vi "Synergy - Position-Position.vi"(10 "Angle for Synergy analysis":dbl[][](array[numeric]), 11 "Position (output)":dbl[][](array[numeric])) -> (2 "Synergy Graph":i32[][](array[numeric]), 3 "Synergy%":i32[][](array[numeric]))   [LabVIEW 2020]
uses:
  <vilib>/Analysis/NI_AALPro.lvlib
panel:
  out "Shoulder Angle Zaxis":dbl[](graph)
  out "WristY-Shoulder Angle Zaxis graph 4":i32[](graph)
  out "WristY-Shoulder AngleZ opposite direction % 4":i32
  out "WristY-Shoulder Angle Zaxis same direction %4":i32
  out "WristY-Shoulder Angle Zaxis graph 3":i32[](graph)
  out "WristY-Shoulder AngleZ opposite direction % 3":i32
  out "WristY-Shoulder Angle Zaxis same direction % 3":i32
  out "WristX-Shoulder Angle Zaxis graph 2":i32[](graph)
  out "WristX-Shoulder Angle Zaxis opposite direction % 2":i32
  out "WristX-Shoulder Angle Zaxis same direction % 2":i32
  out "Wrist Y Tags 2":i32[](array[numeric])
  out "WristY-Elbow Angle Zaxis graph 2":i32[](graph)
  out "WristY-Elbow AngleZ opposite direction % 2":i32
  out "WristY-Elbow Angle Zaxis same direction % 2":i32
  out "WristY-ElbowY graph 2":i32[](graph)
  out "WristY-ElbowY opposite direction % 2":i32
  out "WristY-ElbowY same direction % 2":i32
  out "WristY-ElbowX graph 2":i32[](graph)
  out "WristY-ElbowX opposite direction % 2":i32
  out "WristY-ElbowX same direction % 2":i32
  out "WristY-ShoulderY graph 2":i32[](graph)
  out "WristY-ShouldeY opposite direction % 2":i32
  out "WristY-ShouldeY same direction % 2":i32
  out "WristY-ShoulderX graph 2":i32[](graph)
  out "WristY-ShouldeX opposite direction % 2":i32
  out "WristY- ShoulderX same direction % 2":i32
  out "Elbow Angle Zaxis":dbl[](graph)
  out "WristY-Elbow Angle Zaxis graph":i32[](graph)
  out "WristY-Elbow AngleZ opposite direction %":i32
  out "WristY-Elbow Angle Zaxis same direction %":i32
  out "WristX-Elbow Angle Zaxis graph":i32[](graph)
  out "WristX-Elbow Angle Zaxis opposite direction %":i32
  out "WristX-Elbow Angle Zaxis same direction %":i32
  out "Array 2":i32[](array[numeric])
  out "WristX derivative":dbl[](graph)
  out "WristX":dbl[](graph)
  out "WristX cropped region":dbl[](graph)
  out "WristY-ElbowY graph":i32[](graph)
  out "WristY-ElbowY opposite direction %":i32
  out "WristY-ElbowY same direction %":i32
  out "WristY-ElbowX graph":i32[](graph)
  out "WristY-ElbowX opposite direction %":i32
  out "WristY-ElbowX same direction %":i32
  out "WristY-ShoulderY graph":i32[](graph)
  out "WristY-ShouldeY opposite direction %":i32
  out "WristY-ShouldeY same direction %":i32
  out "WristY-ShoulderX graph":i32[](graph)
  out "WristY-ShouldeX opposite direction %":i32
  out "WristY- ShoulderX same direction %":i32
  out "WristX-ElbowY graph":i32[](graph)
  out "WristX-ElbowY opposite direction %":i32
  out "WristX-ElbowY same direction %":i32
  out "WristX-ElbowX graph":i32[](graph)
  out "WristX-ElbowX opposite direction %":i32
  out "WristX-ElbowX same direction %":i32
  out "WristX-ShoulderY graph":i32[](graph)
  out "WristX-ShouldeY opposite direction %":i32
  out "WristX-ShouldeY same direction %":i32
  out "Shoulder Y to derivate":dbl[](array[numeric])
  out "WristX-ShoulderX graph":i32[](graph)
  out "WristX-ShouldeX opposite direction %":i32
  out "WristX-ShouldeX same direction %":i32
  out "Wrist X to derivate":dbl[](array[numeric])
  out "Wrist X to graph":dbl[](array[numeric])
  out "Shoulder X to derivate":dbl[](array[numeric])
  out "Shoulder X":dbl[](array[numeric])
  out "Wrist Y Tags":i32[](array[numeric])
  out "Wrist X Tags":i32[](array[numeric])
  out "?":dbl[](graph)
  out "Elbow Y":dbl[](graph)
  out "Elbow X":dbl[](graph)
  out "Shoulder Y":dbl[](graph)
  out "?":dbl[](graph)
  # "0 WristX-ShoulderX - same direction\n1 WristX-ShoulderX - opposite direction\n2 WristX-ShoulderY - same direction\n3 - WristX-ShoulderY - opposite direction\n4 WristX-ElbowX - same direction\n5 - WristX-ElbowX - opposite direction\n6 WristX-ElbowY - same direction\n7 - WristX-ElbowY - opposite direction\n8 WristY (up)-ShoulderX - same direction\n9 WristY (up)-ShoulderX - opposite direction\n10 WristY (up)-ShoulderY - same direction\n11 - WristY (up)-ShoulderY - opposite direction\n12 WristY (up)-ElbowX - same direction\n13 - WristY (up)-ElbowX - opposite direction\n14 WristY (up)-ElbowY - same direction\n15 - WristY (up)-ElbowY - opposite direction\n16 WristX-Elbow angle Zaxis - same direction\n17 WristX-Elbow angle Zaxis- opposite direction\n18 WristY (up)-Elbow angle Zaxis - same direction\n19 - WristY (up)-Elbow angle Zaxis - opposite direction\n20 WristY (down)-ShoulderX - same direction\n21 WristY (down)-ShoulderX - opposite direction\n22 WristY (down)-ShoulderY - same direction\n23 - WristY (down)-ShoulderY - opposite direction\n24 WristY (down)-ElbowX - same direction\n25 - WristY (down)-ElbowX - opposite direction\n26 WristY (down)-ElbowY - same direction\n27 - WristY (down)-ElbowY - opposite direction\n28 WristY (down)-Elbow angle Zaxis - same direction\n29 - WristY (down)-Elbow angle Zaxis - opposite direction\n30 WristX-Shoulder angle Zaxis - same direction\n31 WristX-Shoulder angle Zaxis- opposite direction\n32 WristY (up)-Shoulder angle Zaxis - same direction\n33 - WristY (up)-Shoulder angle Zaxis - opposite direction\n34 WristY (down)-Shoulder angle Zaxis - same direction\n35 - WristY (down)-Shoulder angle Zaxis - opposite direction"
  # "wrist Y"
  # "wrist X"
  # "derivative"
  # "derivative"
  # "Shoulder X"
  # "Shoulder Y"
  # "Shoulder Z"
  # "Elbow X"
  # "Elbow Y"
  # "Elbow Z"
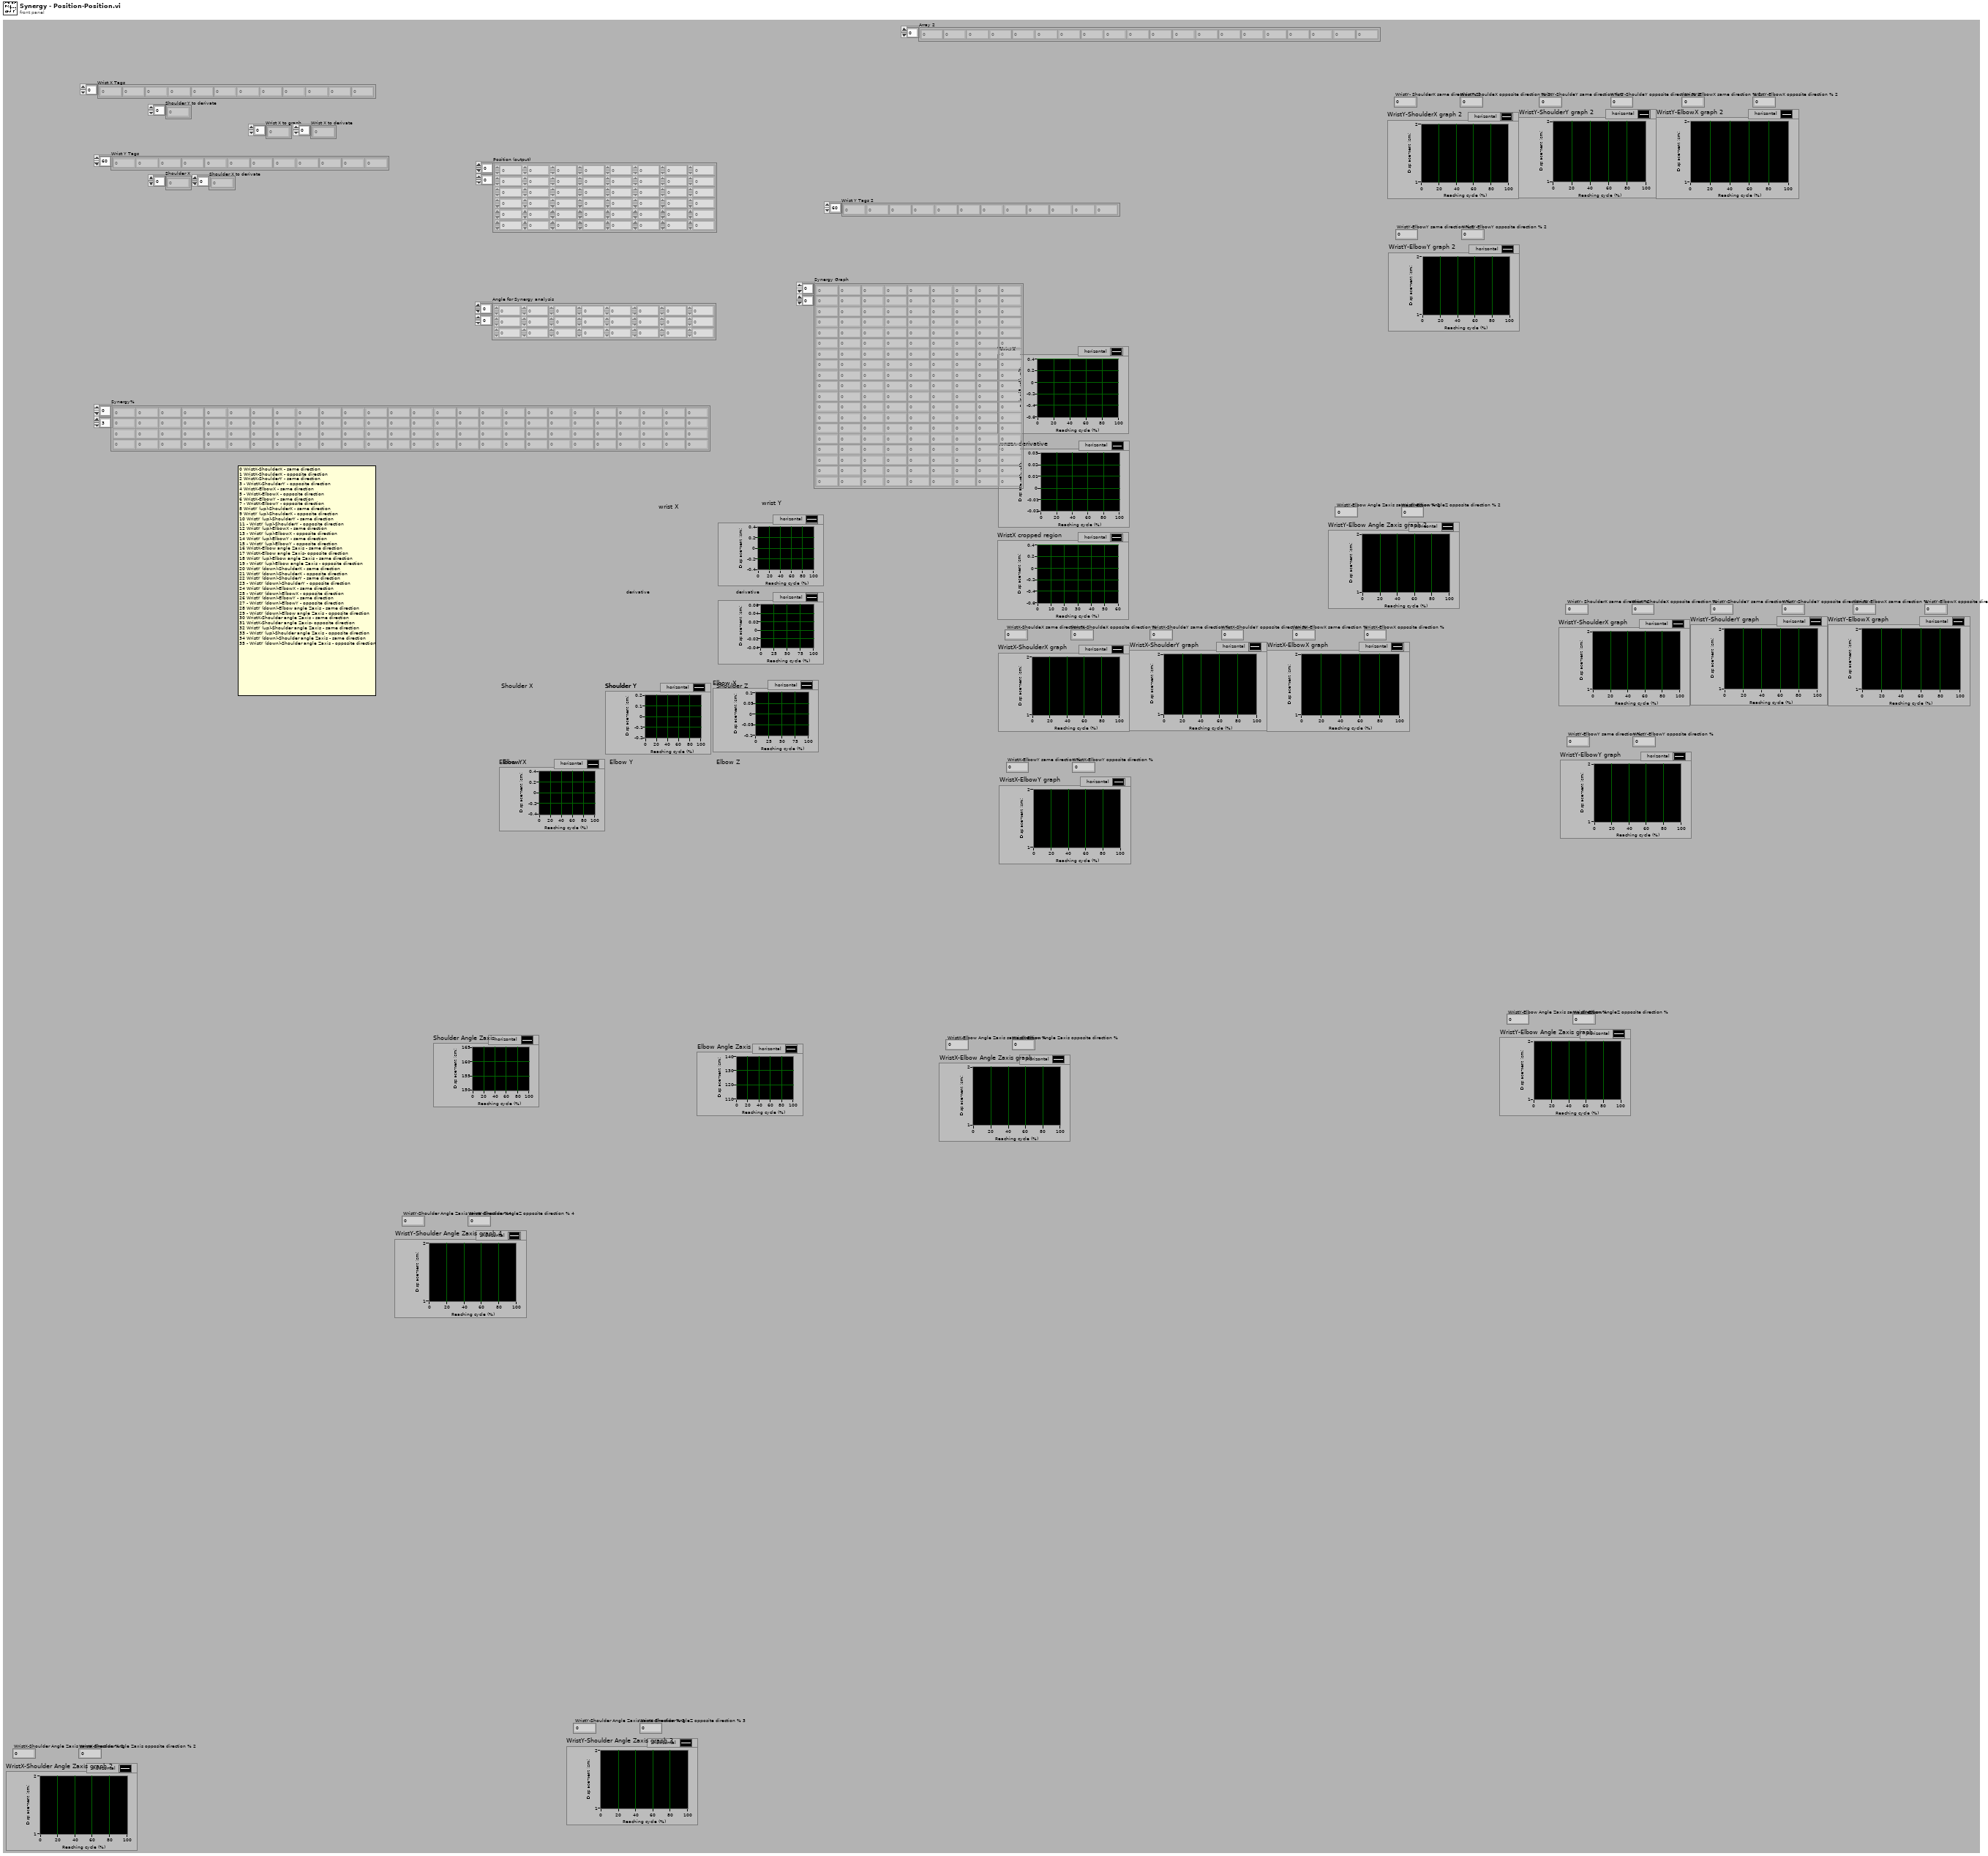
[diagram p1: front panel]
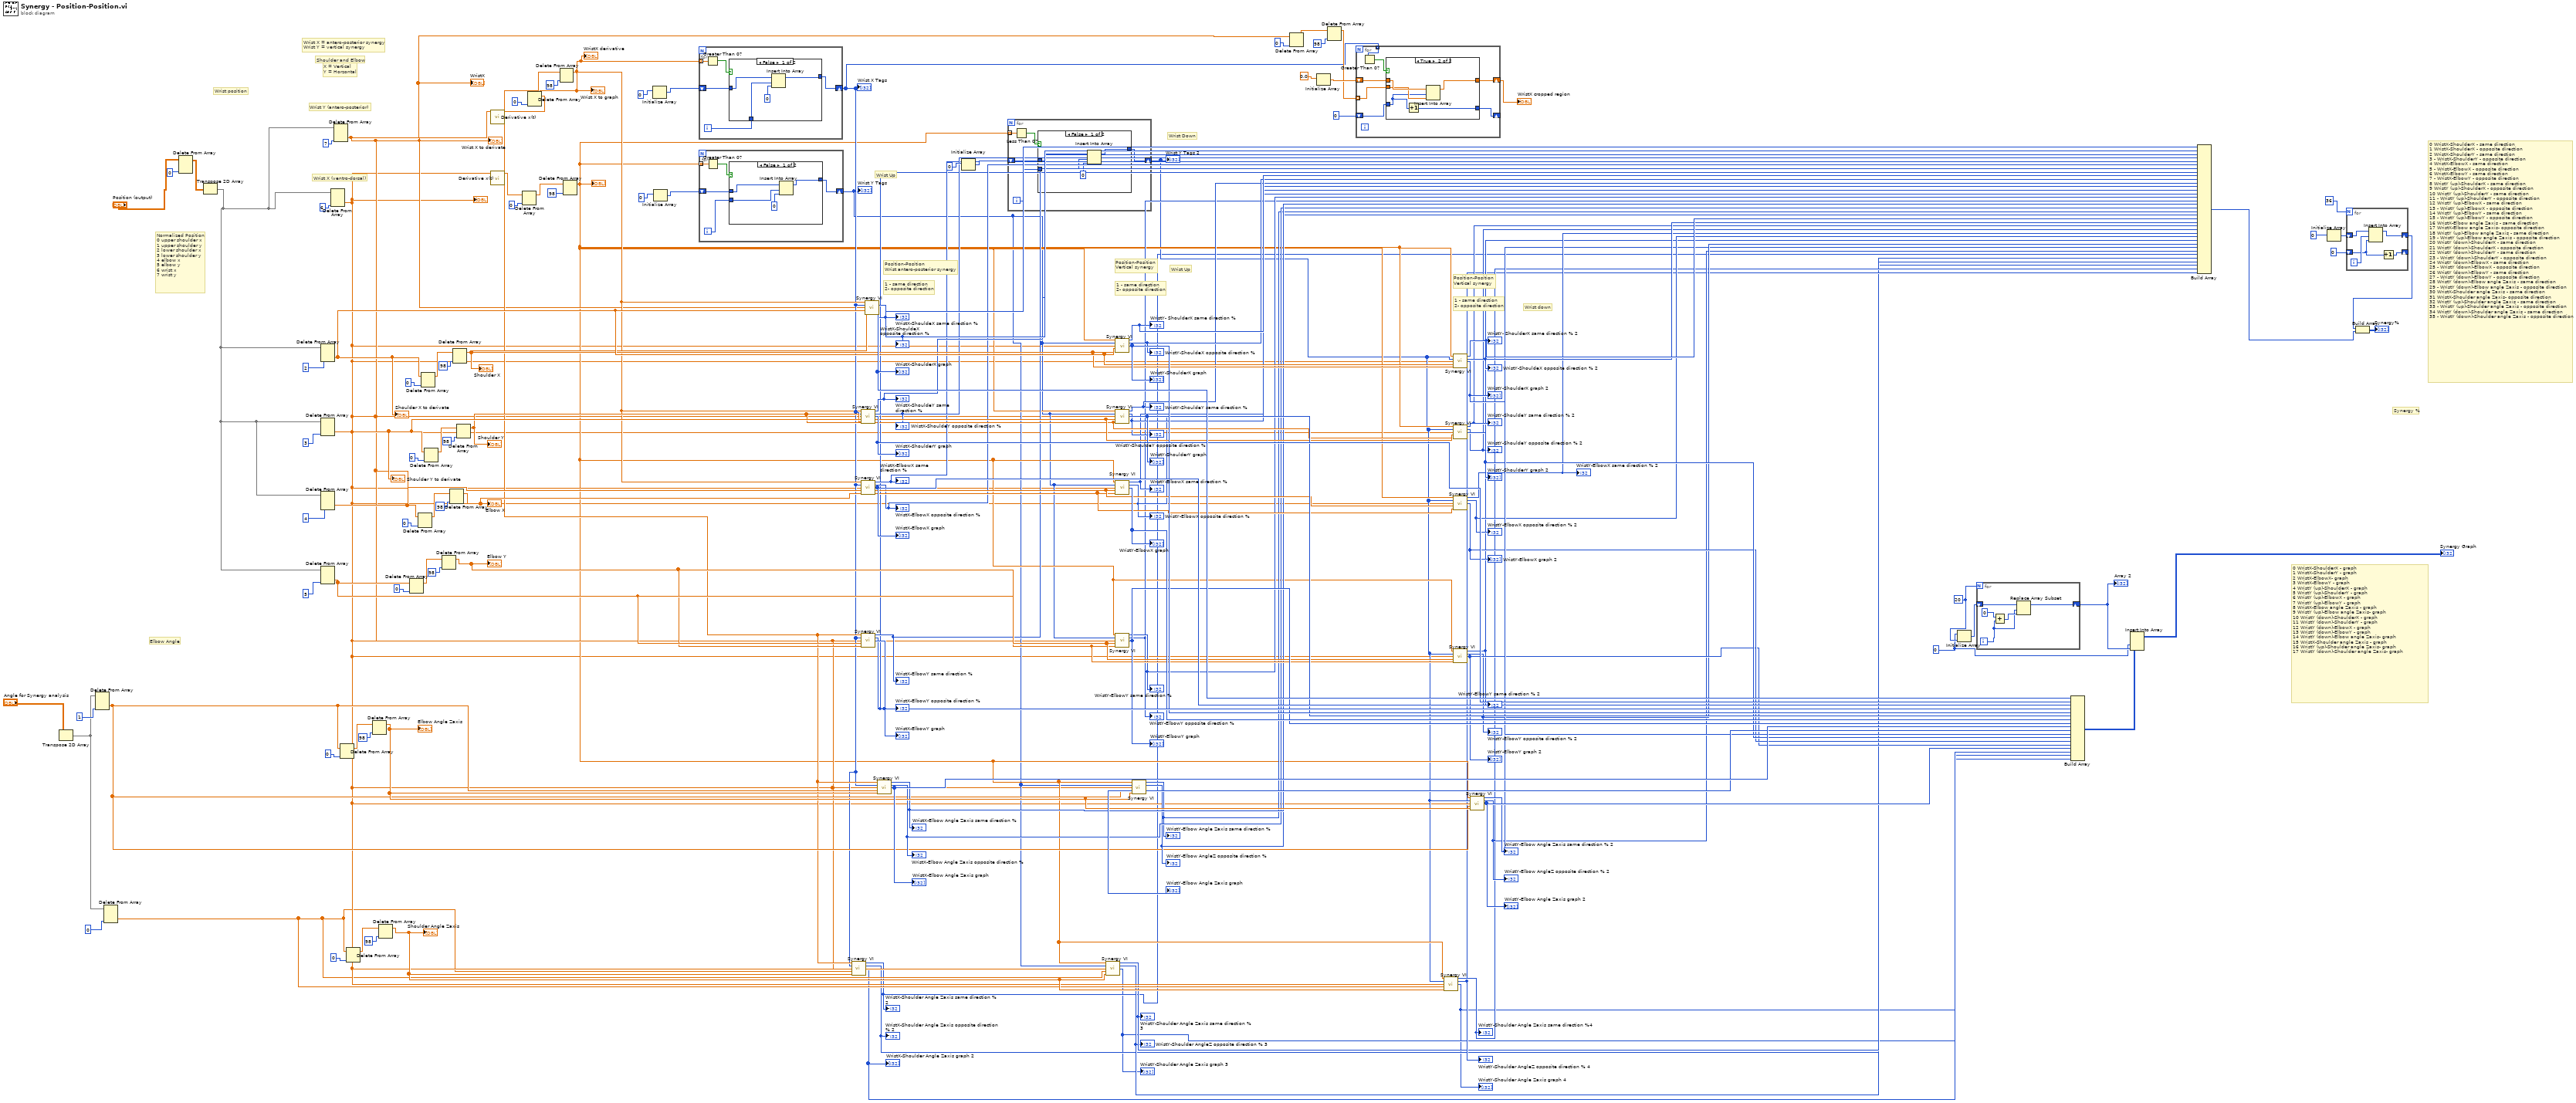
[diagram p0: block diagram]
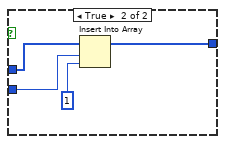
[diagram p2: hidden frame]
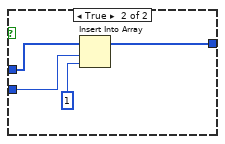
[diagram p4: hidden frame]
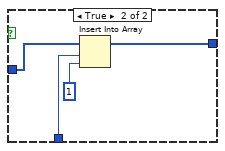
[diagram p5: hidden frame]
diagram:
  w99 = 0
  w101 = 20
  # "Normalized Position\n0 upper shoulder x\n1 upper shoulder y\n2 lower shoulder x\n3 lower shoulder y\n4 elbow x\n5 elbow y\n6 wrist x\n7 wrist y"
  # "Wrist Up"
  # "Wrist down"
  # "Shoulder and Elbow"
  # "Wrist X = antero-posterior synergy\nWrist Y = vertical synergy"
  # "0 WristX-ShoulderX - graph\n1 WristX-ShoulderY - graph\n2 WristX-ElbowX- graph\n3 WristX-ElbowY - graph\n4 WristY (up)-ShoulderX - graph\n5 WristY (up)-ShoulderY - graph\n6 WristY (up)-ElbowX - graph\n7 WristY (up)-ElbowY - graph\n8 WristX-Elbow angle Zaxis - graph\n9 WristY (up)-Elbow angle Zaxis- graph\n10 WristY (down)-ShoulderX - graph\n11 WristY (down)-ShoulderY - graph\n12 WristY (down)-ElbowX - graph\n13 WristY (down)-ElbowY - graph\n14 WristY (down)-Elbow angle Zaxis- graph\n15 WristX-Shoulder angle Zaxis - graph\n16 WristY (up)-Shoulder angle Zaxis- graph\n17 WristY (down)-Shoulder angle Zaxis- graph"
  # "0 WristX-ShoulderX - same direction\n1 WristX-ShoulderX - opposite direction\n2 WristX-ShoulderY - same direction\n3 - WristX-ShoulderY - opposite direction\n4 WristX-ElbowX - same direction\n5 - WristX-ElbowX - opposite direction\n6 WristX-ElbowY - same direction\n7 - WristX-ElbowY - opposite direction\n8 WristY (up)-ShoulderX - same direction\n9 WristY (up)-ShoulderX - opposite direction\n10 WristY (up)-ShoulderY - same direction\n11 - WristY (up)-ShoulderY - opposite direction\n12 WristY (up)-ElbowX - same direction\n13 - WristY (up)-ElbowX - opposite direction\n14 WristY (up)-ElbowY - same direction\n15 - WristY (up)-ElbowY - opposite direction\n16 WristX-Elbow angle Zaxis - same direction\n17 WristX-Elbow angle Zaxis- opposite direction\n18 WristY (up)-Elbow angle Zaxis - same direction\n19 - WristY (up)-Elbow angle Zaxis - opposite direction\n20 WristY (down)-ShoulderX - same direction\n21 WristY (down)-ShoulderX - opposite direction\n22 WristY (down)-ShoulderY - same direction\n23 - WristY (down)-ShoulderY - opposite direction\n24 WristY (down)-ElbowX - same direction\n25 - WristY (down)-ElbowX - opposite direction\n26 WristY (down)-ElbowY - same direction\n27 - WristY (down)-ElbowY - opposite direction\n28 WristY (down)-Elbow angle Zaxis - same direction\n29 - WristY (down)-Elbow angle Zaxis - opposite direction\n30 WristX-Shoulder angle Zaxis - same direction\n31 WristX-Shoulder angle Zaxis- opposite direction\n32 WristY (up)-Shoulder angle Zaxis - same direction\n33 - WristY (up)-Shoulder angle Zaxis - opposite direction\n34 WristY (down)-Shoulder angle Zaxis - same direction\n35 - WristY (down)-Shoulder angle Zaxis - opposite direction"
  # "Wrist Down"
  # "Wrist Up"
  # "1 - same direction\n2- opposite direction"
  # "Position-Position\nVertical synergy"
  # "X = Vertical\nY = Horzontal"
  # "Elbow Angle"
  # "Synergy %"
  # "Wrist X (ventro-dorsal)"
  # "Wrist Y (antero-posterior)"
  # "1 - same direction\n2- opposite direction"
  # "Position-Position\nVertical synergy"
  # "Position-Position\nWrist antero-posterior synergy"
  # "1 - same direction\n2- opposite direction"
  # "Wrist position"
  n1 = Transpose 2D Array(2D array="Angle for Synergy analysis") -> (transposed array=w5:dbl[][])
  n2 = Delete From Array(array=w5, index (col)=1) -> (deleted portion=w36:dbl[])  [unwired: 2 in, 1 out]
  n3 = Delete From Array(array=w5, index (col)=0) -> (deleted portion=w23:dbl[])  [unwired: 2 in, 1 out]
  n4 = Delete From Array(array="Position (output)", index (col)=0) -> (array with subset deleted=w1:dbl[][])  [unwired: 2 in, 1 out]
  n5 = Transpose 2D Array(2D array=w1) -> (transposed array=w89:dbl[][])
  n6 = Delete From Array(array=w89, index (col)=2) -> (deleted portion=w81:dbl[])  [unwired: 2 in, 1 out]
  "Shoulder X to derivate" <- w81
  n7 = Delete From Array(array=w89, index (col)=3) -> (deleted portion=w79:dbl[])  [unwired: 2 in, 1 out]
  "Shoulder Y to derivate" <- w79
  n8 = Delete From Array(array=w89, index (col)=4) -> (deleted portion=w77:dbl[])  [unwired: 2 in, 1 out]
  n9 = Delete From Array(array=w89, index (col)=5) -> (deleted portion=w75:dbl[])  [unwired: 2 in, 1 out]
  n10 = Delete From Array(array=w89, index (col)=6) -> (deleted portion=w24:dbl[])  [unwired: 2 in, 1 out]
  "?" <- w24
  n11 = Delete From Array(array=w89, index (col)=7) -> (deleted portion=w29:dbl[])  [unwired: 2 in, 1 out]
  "Wrist X to derivate" <- w29
  "WristX" <- w29
  n12 = Delete From Array(array=w36, index=0) -> (array with subset deleted=w86:dbl[])  [unwired: 1 in, 1 out]
  n13 = Delete From Array(array=w23, index=0) -> (array with subset deleted=w33:dbl[])  [unwired: 1 in, 1 out]
  n14 = Delete From Array(array=w86, index=98) -> (array with subset deleted=w73:dbl[])  [unwired: 1 in, 1 out]
  "Elbow Angle Zaxis" <- w73
  n15 = Delete From Array(array=w33, index=98) -> (array with subset deleted=w26:dbl[])  [unwired: 1 in, 1 out]
  "Shoulder Angle Zaxis" <- w26
  n16 = Delete From Array(array=w75, index=0) -> (array with subset deleted=w111:dbl[])  [unwired: 1 in, 1 out]
  n17 = Delete From Array(array=w77, index=0) -> (array with subset deleted=w114:dbl[])  [unwired: 1 in, 1 out]
  n18 = Delete From Array(array=w81, index=0) -> (array with subset deleted=w120:dbl[])  [unwired: 1 in, 1 out]
  n19 = Delete From Array(array=w79, index=0) -> (array with subset deleted=w117:dbl[])  [unwired: 1 in, 1 out]
  n20 = Delete From Array(array=w111, index=98) -> (array with subset deleted=w74:dbl[])  [unwired: 1 in, 1 out]
  "Elbow Y" <- w74
  n21 = Delete From Array(array=w114, index=98) -> (array with subset deleted=w76:dbl[])  [unwired: 1 in, 1 out]
  "Elbow X" <- w76
  n22 = Delete From Array(array=w120, index=98) -> (array with subset deleted=w80:dbl[])  [unwired: 1 in, 1 out]
  "Shoulder X" <- w80
  n23 = Delete From Array(array=w117, index=98) -> (array with subset deleted=w78:dbl[])  [unwired: 1 in, 1 out]
  "Shoulder Y" <- w78
  n24 = call <vilib>:"Derivative x(t).vi"("X"=w29) -> ("dX/dt"=w134:dbl[])  [unwired: 9 in, 1 out]
  n25 = call <vilib>:"Derivative x(t).vi"("X"=w24) -> ("dX/dt"=w127:dbl[])  [unwired: 9 in, 1 out]
  n26 = Delete From Array(array=w127, index=0) -> (array with subset deleted=w128:dbl[])  [unwired: 1 in, 1 out]
  n27 = Delete From Array(array=w134, index=0) -> (array with subset deleted=w131:dbl[])  [unwired: 1 in, 1 out]
  n28 = Delete From Array(array=w131, index=98) -> (array with subset deleted=w31:dbl[])  [unwired: 1 in, 1 out]
  "Wrist X to graph" <- w31
  "WristX derivative" <- w31
  n29 = Delete From Array(array=w128, index=98) -> (array with subset deleted=w28:dbl[])  [unwired: 1 in, 1 out]
  "?" <- w28
  n30 = Initialize Array(0) -> (w125:i32[])  [unwired: 1 in]
  n31 = Initialize Array(0) -> (w123:i32[])  [unwired: 1 in]
  n32 = for {
    tunnel: w31 -> [w145] mode=indexing
    shift-right: [w142] -> w30
    shift-left: w125 -> [w143]
    i -> [w141]
    n33 = Greater Than 0?(x=w145) -> (x > 0?=w144:bool)
    n34 = case shown="False" w144 {
      tunnel: w143 -> [w148 w153]
      tunnel: [w147 w152] -> w142
      tunnel: w141 -> [w146 w150]
      frame False {
        n35 = Insert Into Array(array=w148, index=w146, new element=0) -> (w147:i32[])
      }
      frame True {
        n36 = Insert Into Array(array=w153, index=w150, new element=1) -> (w152:i32[])
      }
    }
  }
  "Wrist X Tags" <- w30
  n37 = for {
    tunnel: w28 -> [w158] mode=indexing
    shift-right: [w154] -> w27
    shift-left: w123 -> [w156]
    i -> [w155]
    n38 = Greater Than 0?(x=w158) -> (x > 0?=w157:bool)
    n39 = case shown="False" w157 {
      tunnel: w156 -> [w161 w166]
      tunnel: w155 -> [w159 w163]
      tunnel: [w160 w165] -> w154
      frame False {
        n40 = Insert Into Array(array=w161, index=w159, new element=0) -> (w160:i32[])
      }
      frame True {
        n41 = Insert Into Array(array=w166, index=w163, new element=1) -> (w165:i32[])
      }
    }
  }
  "Wrist Y Tags" <- w27
  n42 = call "Synergy VI.vi"("Wrist X to graph"=w31, "Wrist X Tags"=w30, "Wrist X to derivate"=w29, "Shoulder X to derivate"=w23, "Shoulder X"=w26) -> ("same direction %"=w18:i32, "opposite direction %"=w17:i32, "WristX-ShouldeX graph"=w15:i32[])  [unwired: 8 in]
  "WristX-Shoulder Angle Zaxis same direction % 2" <- w18
  "WristX-Shoulder Angle Zaxis opposite direction % 2" <- w17
  "WristX-Shoulder Angle Zaxis graph 2" <- w15
  n43 = call "Synergy VI.vi"("Wrist X to graph"=w31, "Wrist X Tags"=w30, "Wrist X to derivate"=w29, "Shoulder X to derivate"=w79, "Shoulder X"=w78) -> ("same direction %"=w65:i32, "opposite direction %"=w64:i32, "WristX-ShouldeX graph"=w97:i32[])  [unwired: 8 in]
  "WristX-ShouldeY same direction %" <- w65
  "WristX-ShouldeY opposite direction %" <- w64
  "WristX-ShoulderY graph" <- w97
  n44 = call "Synergy VI.vi"("Wrist X to graph"=w31, "Wrist X Tags"=w30, "Wrist X to derivate"=w29, "Shoulder X to derivate"=w77, "Shoulder X"=w76) -> ("same direction %"=w63:i32, "opposite direction %"=w62:i32, "WristX-ShouldeX graph"=w96:i32[])  [unwired: 8 in]
  "WristX-ElbowX same direction %" <- w63
  "WristX-ElbowX opposite direction %" <- w62
  "WristX-ElbowX graph" <- w96
  n45 = call "Synergy VI.vi"("Wrist X to graph"=w31, "Wrist X Tags"=w30, "Wrist X to derivate"=w29, "Shoulder X to derivate"=w75, "Shoulder X"=w74) -> ("same direction %"=w61:i32, "opposite direction %"=w60:i32, "WristX-ShouldeX graph"=w95:i32[])  [unwired: 8 in]
  "WristX-ElbowY same direction %" <- w61
  "WristX-ElbowY opposite direction %" <- w60
  "WristX-ElbowY graph" <- w95
  n46 = call "Synergy VI.vi"("Wrist X to graph"=w31, "Wrist X Tags"=w30, "Wrist X to derivate"=w29, "Shoulder X to derivate"=w81, "Shoulder X"=w80) -> ("same direction %"=w67:i32, "opposite direction %"=w66:i32, "WristX-ShouldeX graph"=w98:i32[])  [unwired: 8 in]
  "WristX-ShouldeX same direction %" <- w67
  "WristX-ShouldeX opposite direction %" <- w66
  "WristX-ShoulderX graph" <- w98
  n47 = call "Synergy VI.vi"("Wrist X to graph"=w31, "Wrist X Tags"=w30, "Wrist X to derivate"=w29, "Shoulder X to derivate"=w36, "Shoulder X"=w73) -> ("same direction %"=w51:i32, "opposite direction %"=w50:i32, "WristX-ShouldeX graph"=w85:i32[])  [unwired: 8 in]
  "WristX-Elbow Angle Zaxis same direction %" <- w51
  "WristX-Elbow Angle Zaxis opposite direction %" <- w50
  "WristX-Elbow Angle Zaxis graph" <- w85
  n48 = Initialize Array(0) -> (w82:i32[])  [unwired: 1 in]
  n49 = for {
    tunnel: w28 -> [w171] mode=indexing
    shift-right: [w167] -> w25
    shift-left: w82 -> [w169]
    i -> [w168]
    n50 = Less Than 0?(x=w171) -> (x < 0?=w170:bool)
    n51 = case shown="False" w170 {
      tunnel: w169 -> [w174 w179]
      tunnel: w168 -> [w172 w176]
      tunnel: [w173 w178] -> w167
      frame False {
        n52 = Insert Into Array(array=w174, index=w172, new element=0) -> (w173:i32[])
      }
      frame True {
        n53 = Insert Into Array(array=w179, index=w176, new element=1) -> (w178:i32[])
      }
    }
  }
  "Wrist Y Tags 2" <- w25
  n54 = call "Synergy VI.vi"("Wrist X to graph"=w28, "Wrist X Tags"=w27, "Wrist X to derivate"=w24, "Shoulder X to derivate"=w23, "Shoulder X"=w26) -> ("same direction %"=w20:i32, "opposite direction %"=w19:i32, "WristX-ShouldeX graph"=w14:i32[])  [unwired: 8 in]
  "WristY-Shoulder Angle Zaxis same direction % 3" <- w20
  "WristY-Shoulder AngleZ opposite direction % 3" <- w19
  "WristY-Shoulder Angle Zaxis graph 3" <- w14
  n55 = call "Synergy VI.vi"("Wrist X to graph"=w28, "Wrist X Tags"=w27, "Wrist X to derivate"=w24, "Shoulder X to derivate"=w81, "Shoulder X"=w80) -> ("same direction %"=w59:i32, "opposite direction %"=w58:i32, "WristX-ShouldeX graph"=w94:i32[])  [unwired: 8 in]
  "WristY- ShoulderX same direction %" <- w59
  "WristY-ShouldeX opposite direction %" <- w58
  "WristY-ShoulderX graph" <- w94
  n56 = call "Synergy VI.vi"("Wrist X to graph"=w28, "Wrist X Tags"=w27, "Wrist X to derivate"=w24, "Shoulder X to derivate"=w79, "Shoulder X"=w78) -> ("same direction %"=w57:i32, "opposite direction %"=w56:i32, "WristX-ShouldeX graph"=w93:i32[])  [unwired: 8 in]
  "WristY-ShouldeY same direction %" <- w57
  "WristY-ShouldeY opposite direction %" <- w56
  "WristY-ShoulderY graph" <- w93
  n57 = call "Synergy VI.vi"("Wrist X to graph"=w28, "Wrist X Tags"=w27, "Wrist X to derivate"=w24, "Shoulder X to derivate"=w77, "Shoulder X"=w76) -> ("same direction %"=w55:i32, "opposite direction %"=w54:i32, "WristX-ShouldeX graph"=w92:i32[])  [unwired: 8 in]
  "WristY-ElbowX same direction %" <- w55
  "WristY-ElbowX opposite direction %" <- w54
  "WristY-ElbowX graph" <- w92
  n58 = call "Synergy VI.vi"("Wrist X to graph"=w28, "Wrist X Tags"=w27, "Wrist X to derivate"=w24, "Shoulder X to derivate"=w75, "Shoulder X"=w74) -> ("same direction %"=w53:i32, "opposite direction %"=w52:i32, "WristX-ShouldeX graph"=w91:i32[])  [unwired: 8 in]
  "WristY-ElbowY same direction %" <- w53
  "WristY-ElbowY opposite direction %" <- w52
  "WristY-ElbowY graph" <- w91
  n59 = call "Synergy VI.vi"("Wrist X to graph"=w28, "Wrist X Tags"=w27, "Wrist X to derivate"=w24, "Shoulder X to derivate"=w36, "Shoulder X"=w73) -> ("same direction %"=w49:i32, "opposite direction %"=w48:i32, "WristX-ShouldeX graph"=w84:i32[])  [unwired: 8 in]
  "WristY-Elbow Angle Zaxis same direction %" <- w49
  "WristY-Elbow AngleZ opposite direction %" <- w48
  "WristY-Elbow Angle Zaxis graph" <- w84
  n60 = Delete From Array(array=w29, index=0) -> (array with subset deleted=w106:dbl[])  [unwired: 1 in, 1 out]
  n61 = Initialize Array(0.0) -> (w110:dbl[])  [unwired: 1 in]
  n62 = Delete From Array(array=w106, index=98) -> (array with subset deleted=w104:dbl[])  [unwired: 1 in, 1 out]
  n63 = for {
    tunnel: w30 -> [w184] mode=indexing
    shift-right: [w182] -> w103
    shift-left: w110 -> [w183]
    tunnel: w104 -> [w185] mode=indexing
    shift-right: [w180] -> _
    shift-left: 0 -> [w181]
    n64 = Greater Than 0?(x=w184) -> (x > 0?=w186:bool)
    n65 = case shown="True" w186 {
      tunnel: w185 -> [_ w192]
      tunnel: w183 -> [w188 w193]
      tunnel: [w188 w191] -> w182
      tunnel: w181 -> [w187 w190]
      tunnel: [w187 w189] -> w180
      frame False {
      }
      frame True {
        n66 = Increment(x=w190) -> (x+1=w189:i32)
        n67 = Insert Into Array(array=w193, index=w190, new element=w192) -> (w191:dbl[])
      }
    }
  }
  "WristX cropped region" <- w103
  n68 = call "Synergy VI.vi"("Wrist X to graph"=w28, "Wrist X Tags"=w25, "Wrist X to derivate"=w24, "Shoulder X to derivate"=w23, "Shoulder X"=w26) -> ("same direction %"=w22:i32, "opposite direction %"=w21:i32, "WristX-ShouldeX graph"=w13:i32[])  [unwired: 8 in]
  "WristY-Shoulder Angle Zaxis same direction %4" <- w22
  "WristY-Shoulder AngleZ opposite direction % 4" <- w21
  "WristY-Shoulder Angle Zaxis graph 4" <- w13
  n69 = call "Synergy VI.vi"("Wrist X to graph"=w28, "Wrist X Tags"=w25, "Wrist X to derivate"=w24, "Shoulder X to derivate"=w81, "Shoulder X"=w80) -> ("same direction %"=w47:i32, "opposite direction %"=w46:i32, "WristX-ShouldeX graph"=w72:i32[])  [unwired: 8 in]
  "WristY- ShoulderX same direction % 2" <- w47
  "WristY-ShouldeX opposite direction % 2" <- w46
  "WristY-ShoulderX graph 2" <- w72
  n70 = call "Synergy VI.vi"("Wrist X to graph"=w28, "Wrist X Tags"=w25, "Wrist X to derivate"=w24, "Shoulder X to derivate"=w79, "Shoulder X"=w78) -> ("same direction %"=w45:i32, "opposite direction %"=w44:i32, "WristX-ShouldeX graph"=w71:i32[])  [unwired: 8 in]
  "WristY-ShouldeY same direction % 2" <- w45
  "WristY-ShouldeY opposite direction % 2" <- w44
  "WristY-ShoulderY graph 2" <- w71
  n71 = call "Synergy VI.vi"("Wrist X to graph"=w28, "Wrist X Tags"=w25, "Wrist X to derivate"=w24, "Shoulder X to derivate"=w77, "Shoulder X"=w76) -> ("same direction %"=w43:i32, "opposite direction %"=w42:i32, "WristX-ShouldeX graph"=w70:i32[])  [unwired: 8 in]
  "WristY-ElbowX same direction % 2" <- w43
  "WristY-ElbowX opposite direction % 2" <- w42
  "WristY-ElbowX graph 2" <- w70
  n72 = call "Synergy VI.vi"("Wrist X to graph"=w28, "Wrist X Tags"=w25, "Wrist X to derivate"=w24, "Shoulder X to derivate"=w75, "Shoulder X"=w74) -> ("same direction %"=w41:i32, "opposite direction %"=w40:i32, "WristX-ShouldeX graph"=w69:i32[])  [unwired: 8 in]
  "WristY-ElbowY same direction % 2" <- w41
  "WristY-ElbowY opposite direction % 2" <- w40
  "WristY-ElbowY graph 2" <- w69
  n73 = call "Synergy VI.vi"("Wrist X to graph"=w28, "Wrist X Tags"=w25, "Wrist X to derivate"=w24, "Shoulder X to derivate"=w36, "Shoulder X"=w73) -> ("same direction %"=w39:i32, "opposite direction %"=w38:i32, "WristX-ShouldeX graph"=w68:i32[])  [unwired: 8 in]
  "WristY-Elbow Angle Zaxis same direction % 2" <- w39
  "WristY-Elbow AngleZ opposite direction % 2" <- w38
  "WristY-Elbow Angle Zaxis graph 2" <- w68
  n74 = Initialize Array(w99, w101) -> (w102:i32[])
  n75 = for {
    N: w101 -> [_]
    shift-right: [w197] -> w100
    shift-left: w102 -> [w198]
    i -> [w194]
    n76 = Add(x=0, y=w194) -> (x+y=w195:i32)
    n77 = Replace Array Subset(array=w198, new element=w195, index=w194) -> (w197:i32[])
  }
  "Array 2" <- w100
  n78 = Build Array(w98, w97, w96, w95, w94, w93, w92, w91, w85, w84, w72, w71, w70, w69, w68, w15, w14, w13) -> (w90:i32[][])
  n79 = Insert Into Array(array=w90, index (col)=w99, new element=w100) -> (→"Synergy Graph":i32[][])  [unwired: 1 in]
  n80 = Build Array(w67, w66, w65, w64, w63, w62, w61, w60, w59, w58, w57, w56, w55, w54, w53, w52, w51, w50, w49, w48, w47, w46, w45, w44, w43, w42, w41, w40, w39, w38, w18, w17, w20, w19, w22, w21) -> (w7:i32[])
  n81 = Initialize Array(0) -> (w10:i32[])  [unwired: 1 in]
  n82 = for {
    N: 36 -> [_]
    shift-right: [w201] -> w8
    shift-left: w10 -> [w202]
    shift-right: [w199] -> _
    shift-left: 0 -> [w200]
    i -> [w203]
    n83 = Insert Into Array(array=w202, index=w203, new element=w200) -> (w201:i32[])
    n84 = Increment(x=w200) -> (x+1=w199:i32)
  }
  n85 = Build Array(w8, w7) -> (→"Synergy%":i32[][])
